vi "PS_TEMP.vi"(0 "GUID":string) -> (2 "Temp (C)":dbl, 3 "time date":string, 4 "File Path Out":path[](array[path]))   [LabVIEW 2019]
uses:
  5_Controls/PS_CMD_type-def.ctl
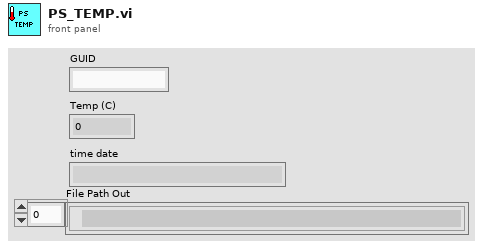
[diagram p1: front panel]
types:
  T1 = typedef "PS_CMD_type-def.ctl" = enum16{"Cond+Temp", "Cond_EIS", "Temp_EIS", "Vwind_MSP", "LongCond", "Cell1_EIS", "Cell2_EIS", "Cell3_EIS"}
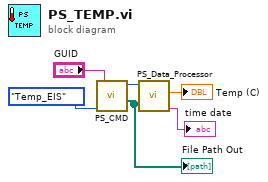
[diagram p0: block diagram]
diagram:
  n1 = call "PS_CMD.vi"(4:PS_CMD_type-def."Temp_EIS", "GUID"="GUID") -> ("File Path Out"=w4:path[], "Enum"=w5:T1)  [unwired: 4 in]
  "File Path Out" <- w4
  n2 = call "PS_Data_Processor.vi"("file path (dialog if empty)"=w4, 11:w5) -> ("time date"=→"time date":string, "Temp (C)"=→"Temp (C)":dbl)  [unwired: 3 in, 5 out]
